vi "Cache Diagnostics.vi"() -> (0 "error out":errorcluster, 3 "Result":bool=TRUE)   [LabVIEW 2013]
doc: "Performs diagnostics on the CPU Cache."
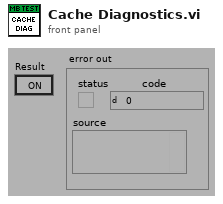
[diagram p1: front panel]
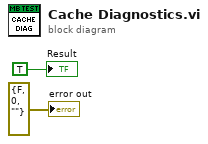
[diagram p0: block diagram]
diagram:
  "error out" <- errorcluster {"status"=FALSE, "code"=0, "source"=""} ("error out")
  "Result" <- TRUE ("PASS/FAIL Flag")
